vi "perform_regex.vi"(10 "regular expression[MAC address format]":string="[0-9A-F]{2}:[0-9A-F]{2}:[0-9A-F]{2}:[0-9A-F]{2}:[0-9A-F]{2}:[0-9A-F]{2}", 11 "input string":string) -> (3 "result":bool)   [LabVIEW 2018]
uses:
  <vilib>/regexp/Match Regular Expression.xnode
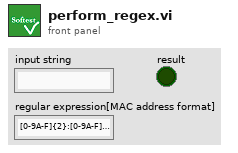
[diagram p1: front panel]
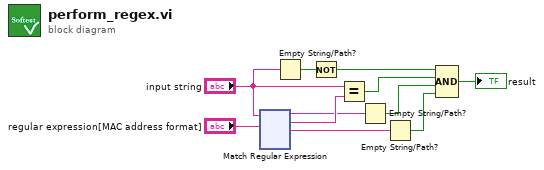
[diagram p0: block diagram]
diagram:
  n1 = xnode "Match Regular Expression"("input string"="input string", "regular expression"="regular expression[MAC address format]") -> ("before match"=w9:string, "whole match"=w10:string, "after match"=w8:string)  [unwired: 4 in, 2 out]
  n2 = Empty String/Path?(string/path="input string") -> (empty?=w3:bool)
  n3 = Not(x=w3) -> (.not. x?=w2:bool)
  n4 = Equal?(x="input string", y=w10) -> (x = y?=w7:bool)
  n5 = Empty String/Path?(string/path=w9) -> (empty?=w6:bool)
  n6 = Empty String/Path?(string/path=w8) -> (empty?=w5:bool)
  n7 = Compound Arithmetic op=AND(w2, w7, w6, w5) -> (→"result":bool)
